vi "jitterArray.vi"(10 "Jitter 2":dbl, 11 "Array":dbl[](array[numeric])) -> (3 "jitteredArray":dbl[](array[numeric]))   [LabVIEW 2013]
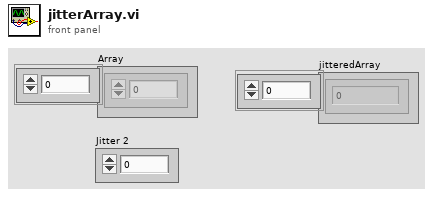
[diagram p1: front panel]
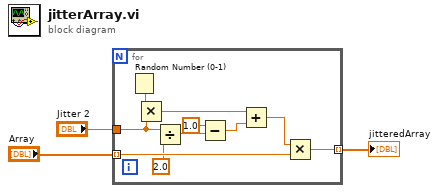
[diagram p0: block diagram]
diagram:
  n1 = for {
    tunnel: "Jitter 2" -> [w5]
    tunnel: "Array" -> [w8] mode=indexing
    tunnel: [w7] -> w1 mode=indexing
    n2 = Random Number (0-1)() -> (number: 0 to 1=w10:dbl)
    n3 = Multiply(x=w10, y=w5) -> (x*y=w12:dbl)
    n4 = Divide(x=w5, y=2.0) -> (x/y=w6:dbl)
    n5 = Subtract(x=1.0, y=w6) -> (x-y=w11:dbl)
    n6 = Add(x=w12, y=w11) -> (x+y=w9:dbl)
    n7 = Multiply(x=w9, y=w8) -> (x*y=w7:dbl)
  }
  "jitteredArray" <- w1
